vi "ROI group vis window-Bring to front.vi"(11 "VI's reference":refnum<vi>) -> ()   [LabVIEW 2020]
uses:
  ROI grouping window/Globals/gl_ROI grp window globals.vi
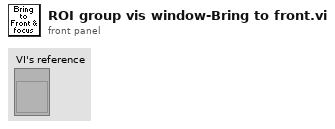
[diagram p1: front panel]
types:
  T1 = enum32{"Invalid", "Standard", "Closed", "Hidden", "Minimized", "Maximized"}
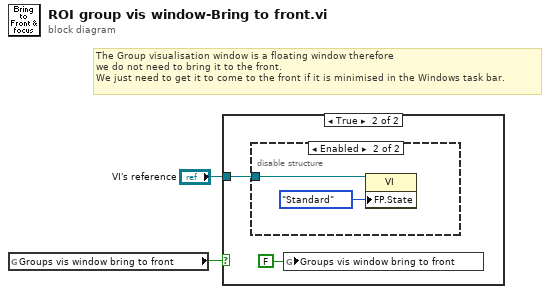
[diagram p0: block diagram]
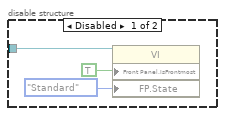
[diagram p3: hidden frame]
diagram:
  # "The Group visualisation window is a floating window therefore\nwe do not need to bring it to the front.\nWe just need to get it to come to the front if it is minimised in the Windows task bar."
  n1 = global read "gl_ROI grp window globals.vi" "Groups vis window bring to front"() -> (w2:bool)
  n2 = case shown="True" w2 {
    tunnel: "VI's reference" -> [_ w3]
    frame False {
    }
    frame True {
      n3 = disable-structure shown="Enabled" {
        disable-tunnel: w3 -> [w5 w8]
        frame Disabled {
          n4 = property class="VI"(reference=w5, "Front Panel.IsFrontmost"=TRUE ("Front Panel Window:Is Frontmost"), "FP.State"=T1."Standard" ("Front Panel Window:State")) -> ()  [unwired: 1 in, 2 out]
        }
        frame Enabled {
          n5 = property class="VI"(reference=w8, "FP.State"=T1."Standard" ("Front Panel Window:State")) -> ()  [unwired: 1 in, 2 out]
        }
      }
      n6 = global write "gl_ROI grp window globals.vi" "Groups vis window bring to front"(FALSE ("Bring to front")) -> ()
    }
  }
